vi "Lab2.vi"() -> ()   [LabVIEW 2015]
panel:
  in  "stop":bool
  out "Numeric":dbl
  out "Meter":dbl(knob) scale=0.0..20.0
  in  "Slide":dbl(slide) scale=0.0..10.0
  in  "Knob":dbl(knob) scale=0.0..10.0
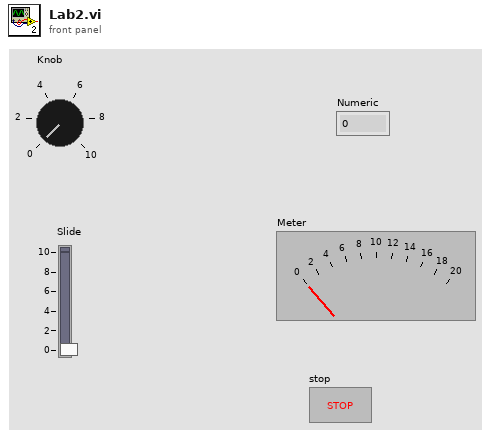
[diagram p1: front panel]
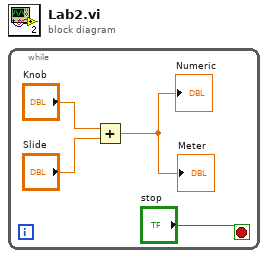
[diagram p0: block diagram]
diagram:
  n1 = while {
    stop <- "stop" stop-if-true
    n2 = Add(x="Knob", y="Slide") -> (x+y=→"Meter" →"Numeric":dbl)
  }
